vi "Thruster8.vi"(1 "Thruster 2":bool, 3 "Truster1":bool, 4 "Floating":bool, 5 "Thruster 3":bool, 6 "Thruster 8":bool, 7 "task in":refnum<k21>, 9 "Thruster 4":bool, 10 "Thruster 7":bool, 12 "Thruster 5":bool, 13 "error in":errorcluster, 14 "Thruster 6":bool) -> (8 "task out":refnum<k21>, 15 "error out":errorcluster)   [LabVIEW 2012]
doc: "I. Description:\nThis example demonstrates how to write values to a digital output channel.\n\nII. Instructions for Running:\n1. Select the digital lines on the DAQ device to be written.\n2. Select a value to write.\nNote: The array control is sized for 8 lines, if using a different amount of lines, change the number of elements in the array to equal the number of lines chosen.\n\nIII. Block Diagram Steps:\n1. Create a Digital Output channel. Use one channel for all lines. You can alternatively use one channel for each line, but then use a different polymorphic version of the DAQmx Write VI.\n2. Call the Start VI to start the task.\n3. Write the digital Boolean array data in a loop until the user hits the stop button or an error occurs. This write VI writes a single sample of digital data on demand, so no timeout is necessary.\n4. Call the Clear Task VI to clear the Task.\n5. Use the popup dialog box to display an error or warning if any.\n\nIV. I/O Connections Overview:\nMake sure your signal output terminals match the Lines I/O Control. In this case wire the item to receive the signal to the first eight digital lines on your DAQ Device."
uses:
  <vilib>/DAQmx/write.llb/DAQmx Write (Digital 1D Bool 1Chan 1Samp).vi
  <vilib>/DAQmx/miscellaneous.llb/DAQmx Fill In Error Info.vi
panel:
  # "Thruster and Air-Floating Control"
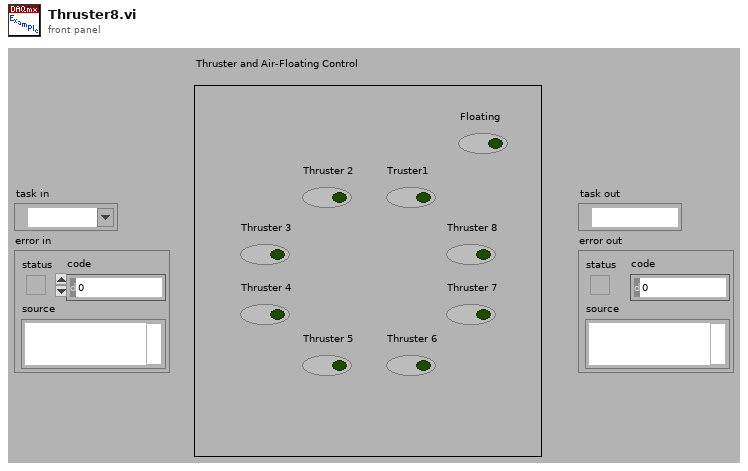
[diagram p1: front panel]
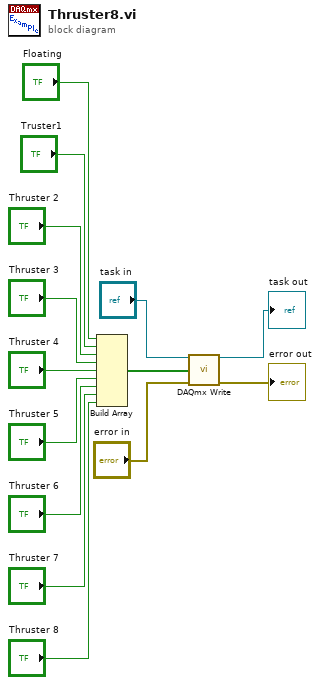
[diagram p0: block diagram]
diagram:
  n1 = Build Array("Floating", "Truster1", "Thruster 2", "Thruster 3", "Thruster 4", "Thruster 5", "Thruster 6", "Thruster 7", "Thruster 8") -> (w3:bool[])
  n2 = call-poly <vilib>:"DAQmx Write.vi"("task/channels in"="task in", "data"=w3, "error in"="error in") -> ("task out"=→"task out":refnum<k21>, "error out"=→"error out":errorcluster)  [unwired: 10 in, 1 out]
